vi "Check Path Status.vi"(11 "Path In":path) -> (2 "File Path Status":T1 caption="Enum 3", 3 "Path Out":path)   [LabVIEW 2024]
uses:
  TypeDef/File Path Status.ctl
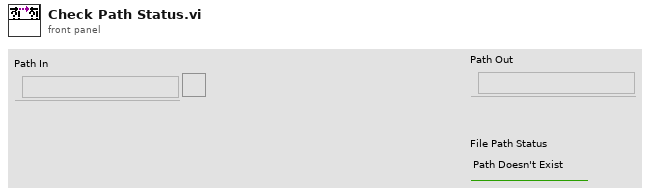
[diagram p1: front panel]
types:
  T1 = typedef "File Path Status.ctl" = enum16{"Path Doesn't Exist", "Path Exist", "Empty Path", "Not A Path"}
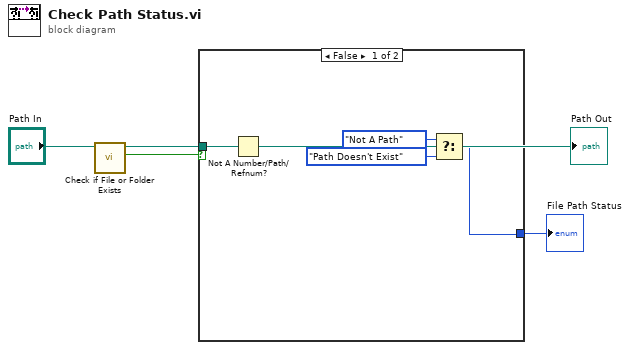
[diagram p0: block diagram]
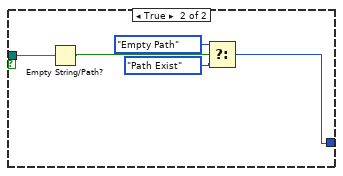
[diagram p2: hidden frame]
diagram:
  n1 = call <vilib>:"Check if File or Folder Exists.vi"("path"="Path In") -> ("file or folder exists?"=w3:bool, "dup path"=w1:path)  [unwired: 8 in, 1 out]
  "Path Out" <- w1
  n2 = case shown="False" w3 {
    tunnel: [w8 w10] -> w2
    tunnel: w1 -> [w9 w14]
    frame False {
      n3 = Not A Number/Path/Refnum?(number/path/refnum=w9) -> (NaN/Path/Refnum?=w7:bool)
      n4 = Select(t=File_Path_Status."Not A Path" ("f"), s=w7, f=File_Path_Status."Path Doesn't Exist" ("File Path Status")) -> (s? t:f=w8:T1)
    }
    frame True {
      n5 = Empty String/Path?(string/path=w14) -> (empty?=w12:bool)
      n6 = Select(t=File_Path_Status."Empty Path" ("File Path Status"), s=w12, f=File_Path_Status."Path Exist" ("File Path Status")) -> (s? t:f=w10:T1)
    }
  }
  "File Path Status" <- w2
